vi "SearchCommandGUI.vi"() -> ()   [LabVIEW 2009, in "DelayGenerator.lvlib"]
uses:
  DelayGenerator.lvlib
panel:
  in  "Turn around":enum16{"In place", "Zero", "Half"}(ring)
  in  "stop":bool
  out "Current Offset":dbl[unit](graph)
  in  "Sign":dbl=1.0
  in  "Growth":dbl[unit]=0.00019999999999999998
  in  "Step":dbl[unit]=1.9999999999999998e-05
  in  "Start Offset":dbl[unit]=-0.9908 format="%.6g"
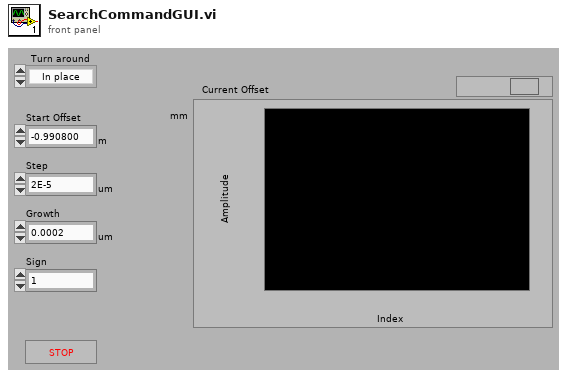
[diagram p1: front panel]
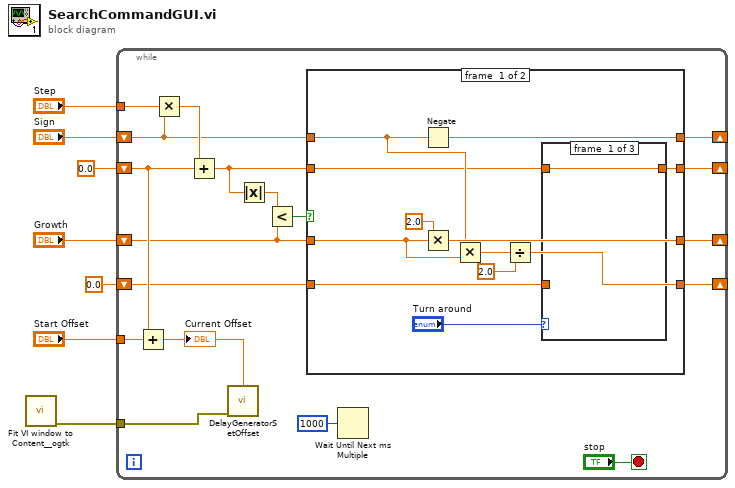
[diagram p0: block diagram]
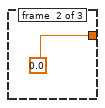
[diagram p2: hidden frame]
diagram:
  n1 = call <userlib>:"Fit VI window to Content__ogtk.vi"() -> ("error out"=w1:errorcluster)  [unwired: 6 in, 1 out]
  n2 = while {
    tunnel: "Step" -> [w24]
    shift-right: [w15] -> _
    shift-left: dbl[unit] 0.0 ("Start Offset") -> [w22]
    shift-right: [w16] -> _
    shift-left: "Sign" -> [w17]
    tunnel: "Start Offset" -> [w21]
    shift-right: [w13] -> _
    shift-left: "Growth" -> [w14]
    shift-right: [w11] -> _
    shift-left: dbl[unit] 0.0 ("Growth") -> [w12]
    tunnel: w1 -> [w8]
    stop <- "stop" stop-if-true
    n3 = Add(x=w22, y=w21) -> (x+y=w9:dbl[unit])
    "Current Offset" <- w9
    n4 = Multiply(x=w24, y=w17) -> (x*y=w23:dbl[unit])
    n5 = Add(x=w23, y=w22) -> (x+y=w18:dbl[unit])
    n6 = call "DelayGeneratorSetOffset.vi"("Offset"=w9, "error in (no error)"=w8) -> ()  [unwired: 7 in, 1 out]
    n7 = Absolute Value(x=w18) -> (abs(x)=w20:dbl[unit])
    n8 = Less?(x=w20, y=w14) -> (x < y?=w19:bool)
    n9 = case shown="False" w19 {
      tunnel: w18 -> [w27 w43]
      tunnel: w17 -> [w33 w44]
      tunnel: [w31 w44] -> w16
      tunnel: [w28 w43] -> w15
      tunnel: w14 -> [w35 w42]
      tunnel: [w37 w42] -> w13
      tunnel: w12 -> [w29 w41]
      tunnel: [w32 w41] -> w11
      frame #0 {
        n10 = Negate(x=w33) -> (-x=w31:dbl)
        n11 = Multiply(x=2.0, y=w35) -> (x*y=w37:dbl[unit])
        n12 = Multiply(x=w33, y=w35) -> (x*y=w34:dbl[unit])
        n13 = Divide(x=w34, y=2.0) -> (x/y=w32:dbl[unit])
        n14 = case shown="\"Half\"" "Turn around" {
          tunnel: w29 -> [_ _ w40]
          tunnel: [w38 dbl[unit] 0.0 ("Growth") w40] -> w28
          tunnel: w27 -> [w38 _ _]
          frame #0 {
          }
          frame #1 {
          }
          frame #2 {
          }
        }
      }
      frame #1 {
      }
    }
    n15 = Wait Until Next ms Multiple(millisecond multiple=u32 1000) -> ()  [unwired: 1 out]
  }
